vi "Sequential State Machine.vi"(6 "Base State":i32, 8 "Change State":i32, 9 "Old State":i32, 10 "Change Condition":bool, 11 "Button Press":bool) -> (3 "Out State":i32)   [LabVIEW 2014]
doc: "This VI will go to the <b>Base State</b> upon the button press, and wait on the change condition before going to the <b>Change State</b>.\n\nThis vi is meant to in a control loop for a given state, other vi's may change the values of the state in the sequence however this will override the stored control data."
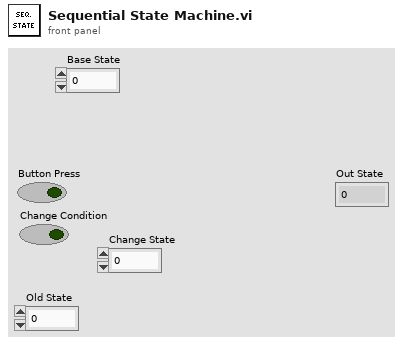
[diagram p1: front panel]
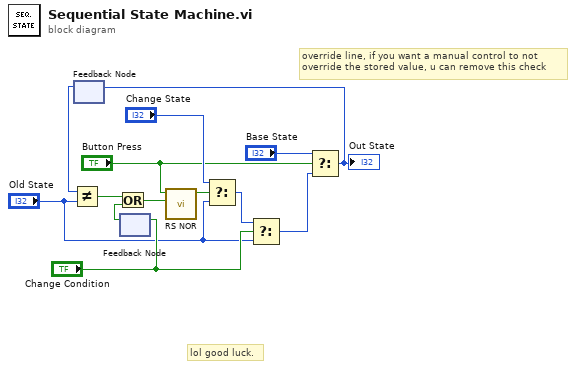
[diagram p0: block diagram]
diagram:
  # "override line, if you want a manual control to not \noverride the stored value, u can remove this check"
  # "lol good luck."
  n1 = feedback #1() -> (w5:i32)  [unwired: 1 in]
  n2 = Not Equal?(x=w5, y="Old State") -> (x != y?=w3:bool)
  n3 = feedback-in #2("Change Condition") -> ()
  n4 = feedback #2() -> (w2:bool)  [unwired: 1 in]
  n5 = Or(x=w3, y=w2) -> (x .or. y?=w1:bool)
  n6 = call "RS NOR.vi"("Reset"=w1, "Set"="Button Press") -> ("Out"=w13:bool)  [unwired: 9 in]
  n7 = Select(t="Change State", s=w13, f="Old State") -> (s? t:f=w11:i32)
  n8 = Select(t=w11, s="Change Condition", f="Old State") -> (s? t:f=w7:i32)
  n9 = Select(t="Base State", s="Button Press", f=w7) -> (s? t:f=w6:i32)
  "Out State" <- w6
  n10 = feedback-in #1(w6) -> ()
